vi "Send Immediate Trigger.vi"(8 "error in (no error)":errorcluster, 10 "Trigger System (0: Acquisition)":u16(ring) items=["Acquisition", "External Logging", "Transient"], 11 "VISA resource name":refnum<visa-resource-name>) -> (0 "error out":errorcluster, 3 "VISA resource name out":refnum<visa-resource-name>)   [LabVIEW 2019, in "Agilent N7976A.lvlib"]
doc: "Initiate commands initialize the trigger system. This moves the trigger system from the \"idle\" state to the \"wait-for- trigger\" state; which enables the instrument to receive triggers. An event on the selected trigger source causes the trigger to occur.\n\nThis sends an Immediate trigger and will cause it to arm immediately REGARDLESS of what trigger setting is currently set.\n\nNote:\nUse this VI only with other low-level VIs. The high-level VIs automatically incorporate this functionality. This VI does not check the instrument status."
uses:
  <instrlib>/Agilent N7976A/Agilent N7976A.lvlib
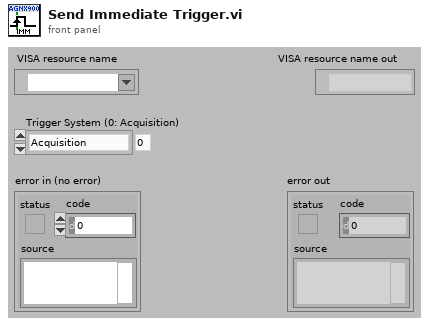
[diagram p1: front panel]
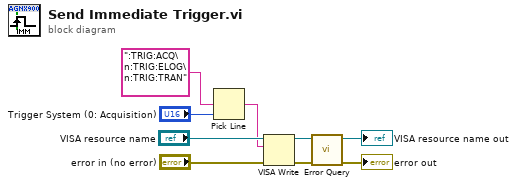
[diagram p0: block diagram]
diagram:
  n1 = Pick Line(multi-line string=":TRIG:ACQ\n:TRIG:ELOG\n:TRIG:TRAN", line index="Trigger System (0: Acquisition)") -> (output string=w3:string)  [unwired: 1 in]
  n2 = VISA Write(VISA resource name="VISA resource name", write buffer=w3, error in (no error)="error in (no error)") -> (VISA resource name out=w6:refnum<visa-resource-name>, error out=w7:errorcluster)  [unwired: 1 out]
  n3 = call <instrlib>:"Error Query.vi"("error in (no error)"=w7, "VISA resource name"=w6) -> ("error out"=→"error out":errorcluster, "VISA resource name out"=→"VISA resource name out":refnum<visa-resource-name>)  [unwired: 6 in, 2 out]
